vi "Pre Test Konfig.vi"() -> ()   [LabVIEW 2020, in "EPA 1065.lvlib" / "Pre-test verification 1065-520.lvlib"]
uses:
  Pre-test verification 1065-520.lvlib
  Allgemein/allgemeine Sub-VIs.lvlib
  Seiten/FT-IR/FT-IR.lvlib
  Seiten/FT-IR/FGV FT-IR Gasliste Aktionen.ctl
  Messdaten/Aktionen FGV Messdaten.ctl
  Messdaten/Messdaten.lvlib
  Seiten/Grafik/Grafik.lvlib
  Funktionstasten/Funktionstasten.lvlib
  Funktionstasten/Funktionstasten-Aktion.ctl
  Funktionstasten/Zustaende.ctl
  Seiten/Gaszuordnung AO/Gaszuordnung AO.lvlib
  Seiten/Gaszuordnung AO/FGV Gaszuordnung Grenzen&Einheit Aktion.ctl
  EPA 1065.lvlib
  Allgemeine VIs/Aktion Wertaenderung Gasliste.ctl
  Allgemeine VIs/Aktion Test Status.ctl
  Sprachverwaltung/Sprachverwaltung.lvlib
  Sprachverwaltung/FGV Aktion Tabelle zerlegen.ctl
  Aktion FGV Pre Test Daten.ctl
  Aktion FGV Pre Test Zustandsautomat.ctl
  PDF_Interface/PDF Interface Helper/PDFResultPictures.ctl
  PDF_Interface/PDF Interface Helper/PDF Interface Helper.lvlib
  T90 1065-308/Ergebnis.ctl
  T90 1065-308/T90 Test 1065-308.lvlib
  Visualisierungs Elemente/Zahlen-Ausgabefeld.ctl
  Pre Konfig Daten.ctl
  Modus Pre Test.ctl
panel:
  out "Ergebnis PDF FALSE":T1 caption="Ergebnis 2"
  out "Ergebnis PDF TRUE":T1 caption="Ergebnis 1"
  in  "Gasliste geändert":bool
  in  "Registerkarte":enum32{"Settings", "PRE Test", "Result"}(tab)
  in  "Pre Konfig Daten":T2={"Bearbeiter:"="", "Messgerät:"="", "Seriennummer:"="", "Modus"=0, "Pfad:"=path "D:/IAG_Data/Log", "Textname:"="", "N2 Aufschaltzeit:"=120.0, "Flow weighted mean:"=0.0} {"Flow weighted mean:" min=10.0; "N2 Aufschaltzeit:" min=10.0; "Modus" items=["Messen", "CalGas zu Entnahme"]}
  in  "Speichern":bool
  out "Einheit":string
  out "Komponente":string caption="Komponente:"
  out "Status":string
  out "Pre":waveform(dbl)(graph)
  in  "Test Start":bool
  in  "Abbrechen":bool
  out "Istwert":T4 caption="Istwert:" format="%.2f"
  out "Mwert":sgl format="%.3f"
  out "PMwert":sgl format="%.3f"
  out "Einheit Genauigkeit 2":string
  out "Ergebnis 1":T1
  out "Ergebnis THC":string
  out "Grenze":string caption="Grenzwert:"
  out "Einheit Genauigkeit":string
  out "Pre Result":waveform(dbl)(graph) caption="Pre"
  in  "Print PDF":bool caption="Abbrechen"
  out "Komponente 2":string caption="Komponente:"
  # "Pre Test Verification EPA CRF40 §1065.520"
  # "Allgemeine Einstellungen"
  # "Protokoll Einstellung"
  # "ppm"
  # "sec."
  # "±"
  # "x"
  # "Grenzwerte"
  # "Ergebnis"
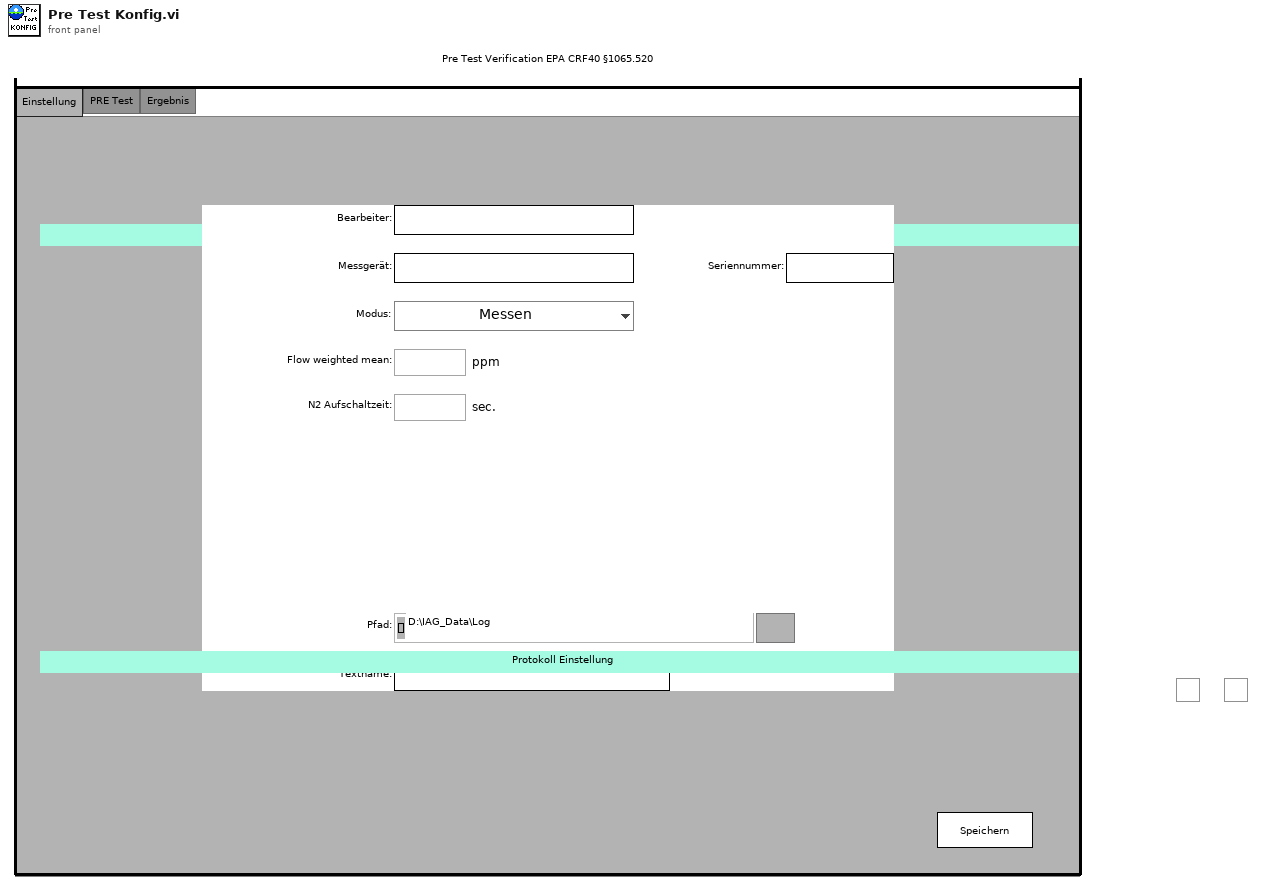
[diagram p1: front panel]
types:
  T1 = typedef "EPA 1065.lvlib/T90 Test 1065-308.lvlib/Ergebnis.ctl" = bool
  T2 = typedef "EPA 1065.lvlib/Pre-test verification 1065-520.lvlib/Pre Konfig Daten.ctl" = cluster{"Bearbeiter:":string, "Messgerät:":string, "Seriennummer:":string, "Modus":T3, "Pfad:":path, "Textname:":string, "N2 Aufschaltzeit:":dbl, "Flow weighted mean:":dbl}
  T3 = typedef "EPA 1065.lvlib/Pre-test verification 1065-520.lvlib/Modus Pre Test.ctl" = u16
  T4 = typedef "Zahlen-Ausgabefeld.ctl" = sgl
  T5 = typedef "EPA 1065.lvlib/Pre-test verification 1065-520.lvlib/Aktion FGV Pre Test Daten.ctl" = enum16{"lesen", "Konfig Daten", "PDF einstellen", "laden", "speichern", "Werte schreiben", "Auswerten"}
  T6 = typedef "EPA 1065.lvlib/Pre-test verification 1065-520.lvlib/Aktion FGV Pre Test Zustandsautomat.ctl" = enum16{"init", "lesen", "leerlauf", "0-Gas aufschalten", "0-Gas abwarten", "aufzeichnen", "fertig", "abbrechen"}
  T7 = typedef "Gaszuordnung AO.lvlib/FGV Gaszuordnung Grenzen&Einheit Aktion.ctl" = enum16{"Lesen", "Schreiben Min", "Schreiben Max", "Laden", "Speichern"}
  T8 = typedef "FT-IR.lvlib/FGV FT-IR Gasliste Aktionen.ctl" = enum16{"lesen", "Gasliste FT-IR", "Gasliste ausgelesen", "laden", "speichern", "löschen"}
  T9 = typedef "Sprachverwaltung.lvlib/FGV Aktion Tabelle zerlegen.ctl" = enum16{"laden", "vereinzeln", "speichern"}
  T10 = typedef "Messdaten.lvlib/Aktionen FGV Messdaten.ctl" = enum16{"lesen", "schreiben", "löschen", "Mittelwerte", "Komponente"}
  T11 = typedef "PDF Interface.lvlib/PDF Interface Helper.lvlib/PDFResultPictures.ctl" = cluster{"Yes Ctl Refnum":refnum<vi>, "No Ctl Refnum":refnum<vi>}
  T12 = typedef "String - Ausgabefeld.ctl" = string
  T13 = typedef "EPA 1065.lvlib/Aktion Wertaenderung Gasliste.ctl" = enum16{"Init", "lesen", "Gasliste geändert", "ARN inaktiv", "LEAK inaktiv", "Interference 366 inaktiv", "T90 inaktiv", "Interference 375 inaktiv", "Chiller inaktiv", "FID O2 inaktiv", "FID Opti inaktiv", "Drift inaktiv", "Pre Test inaktiv", "LinV2 inaktiv", "HovaCAL Interference inaktiv"}
  T14 = typedef "EPA 1065.lvlib/Aktion Test Status.ctl" = enum16{"init", "lesen", "prüfen", "Interference 366", "Interference 375", "Chiller läuft", "Drift läuft", "Pre Test läuft", "FID Optimization läuft", "FID Interference läuft", "HovaCAL Interference", "LinV2"}
  T15 = typedef "Funktionstasten.lvlib/Zustaende.ctl" = enum16{"Standby", "Pause", "Eco", "Messen", "Kalibrieren", "Spülen Filter", "Spülen Leitung", "Umgebungsluft", "0-Gas", "Cal-Gas", "CG zu PNS", "-------------", "Init 1", "Init 2", "Init 3", "Init 4", "Messen vorbereiten", "Messen durchführen", "Exit"}
  T16 = typedef "Funktionstasten.lvlib/Funktionstasten-Aktion.ctl" = enum16{"Initialisieren", "Zustand setzen", "Taste gedrückt", "Fehler speichern", "Lesen", "Manuell", "Remote", "Bitparallel", "Samplepoint", "Zeit Prüfen", "reset Umschalten"}
  T17 = typedef "EPA 1065.lvlib/Pre-test verification 1065-520.lvlib/Pre Werte.ctl" = cluster{"THC Wert":dbl, "Berechnetes Limit":dbl, "Bestanden":bool}
  T18 = typedef "EPA 1065.lvlib/Aktive Tests Cluster.ctl" = cluster{"ANR läuft":bool, "T90 läuft":bool, "Leak läuft":bool, "Interference 366 läuft":bool, "Interference 375 läuft":bool, "Chiller läuft":bool, "FID Interference läuft":bool, "FID optimization läuft":bool, "Drift läuft":bool, "Pre-test läuft":bool, "HovaCAL Interference läuft":bool, "LinV2 läuft":bool}
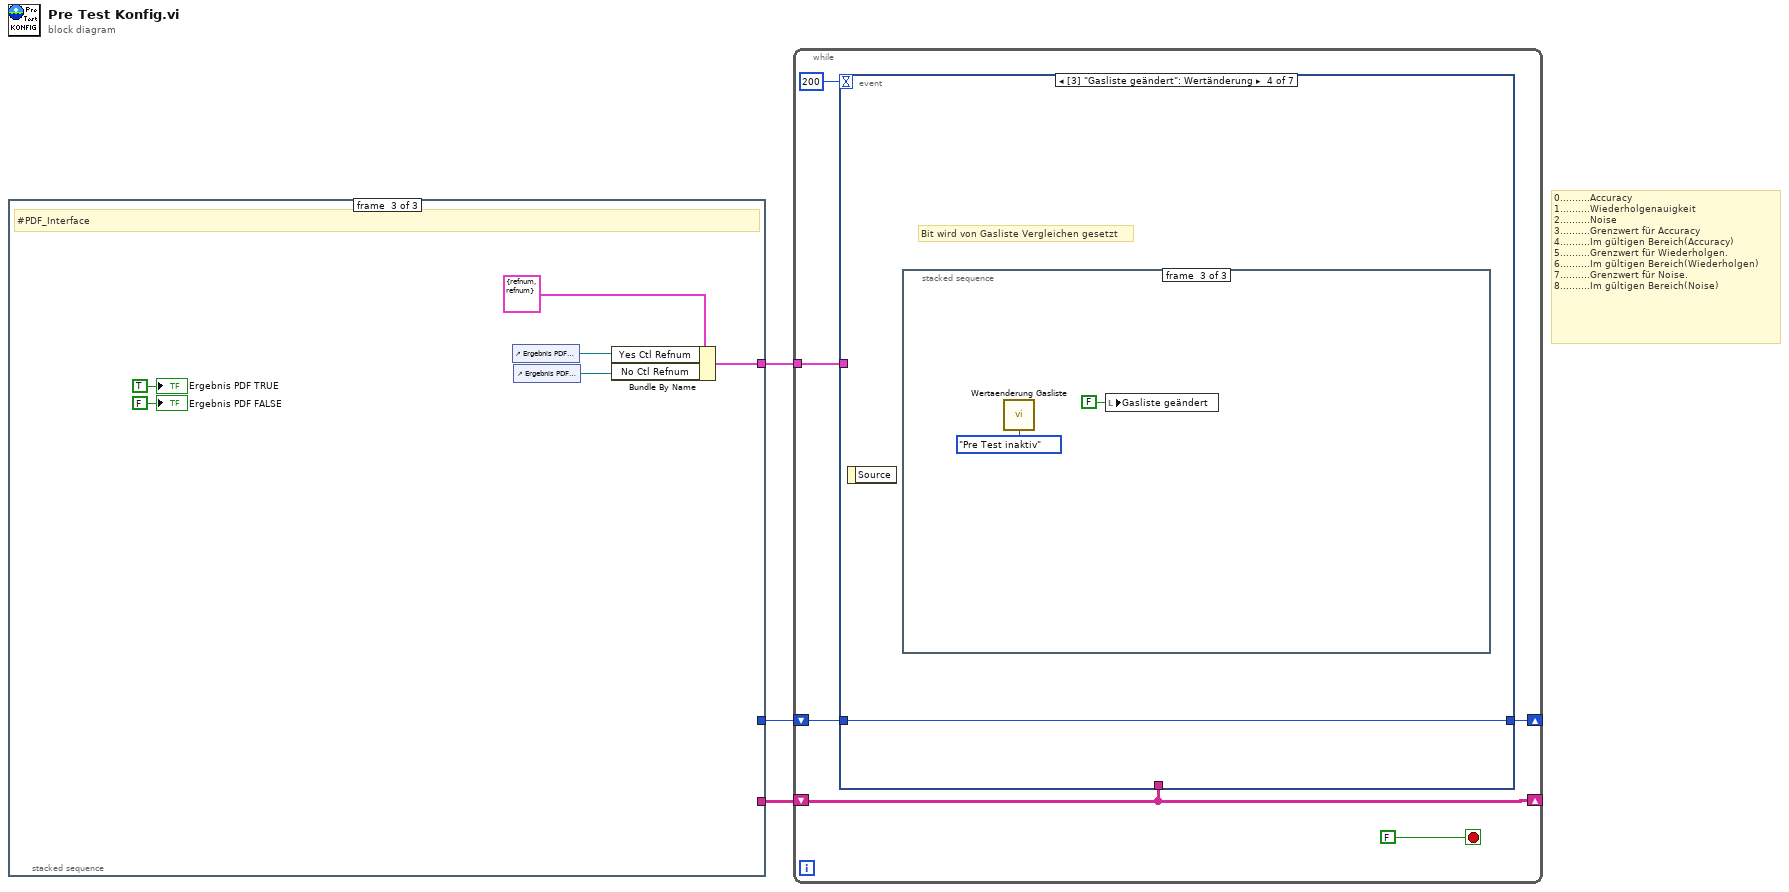
[diagram p0: block diagram]
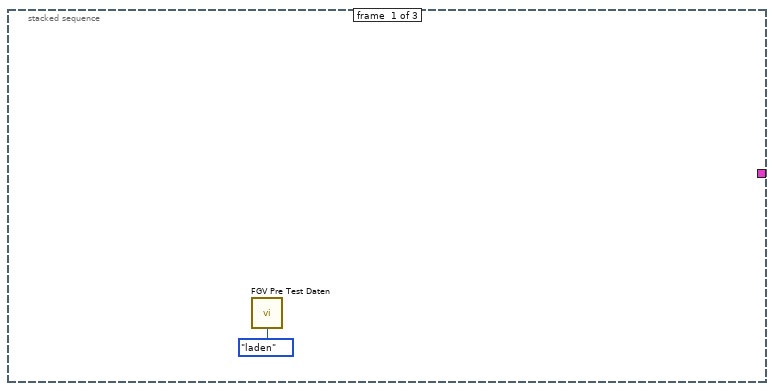
[diagram p2: hidden frame]
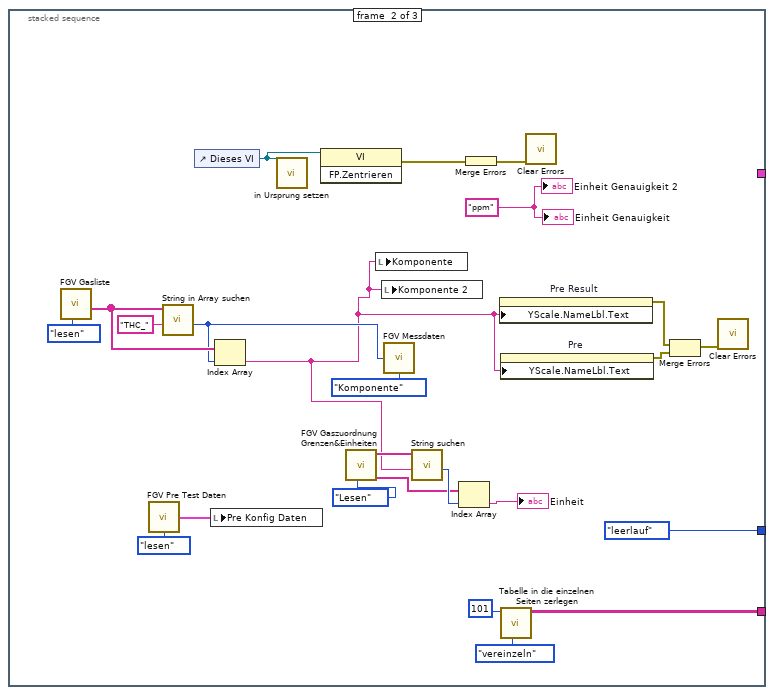
[diagram p3: hidden frame]
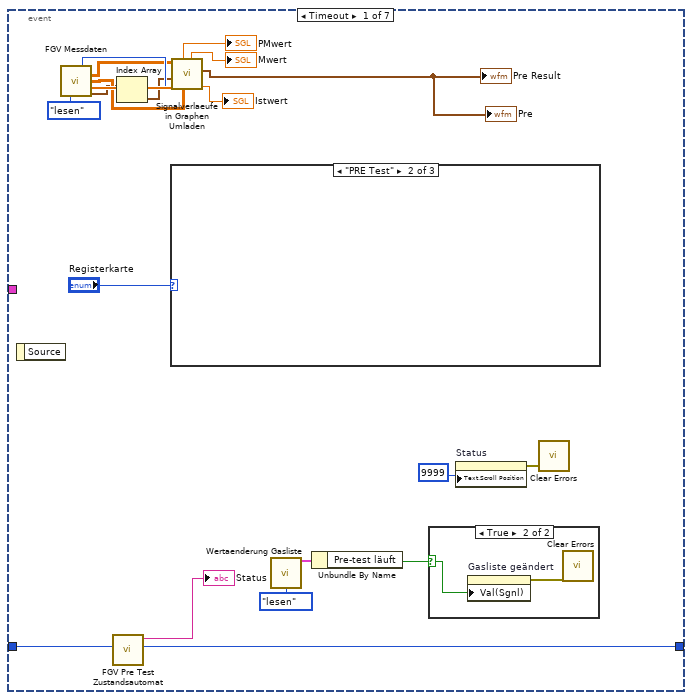
[diagram p4: hidden frame]
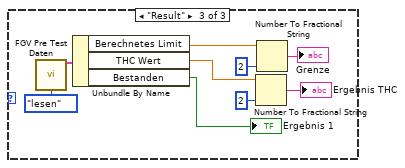
[diagram p6: hidden frame]
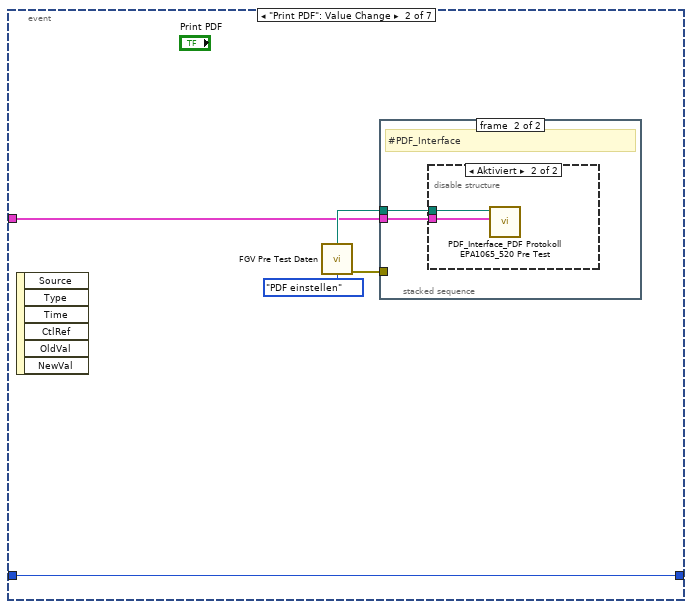
[diagram p8: hidden frame]
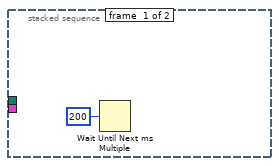
[diagram p9: hidden frame]
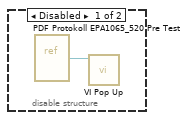
[diagram p10: hidden frame]
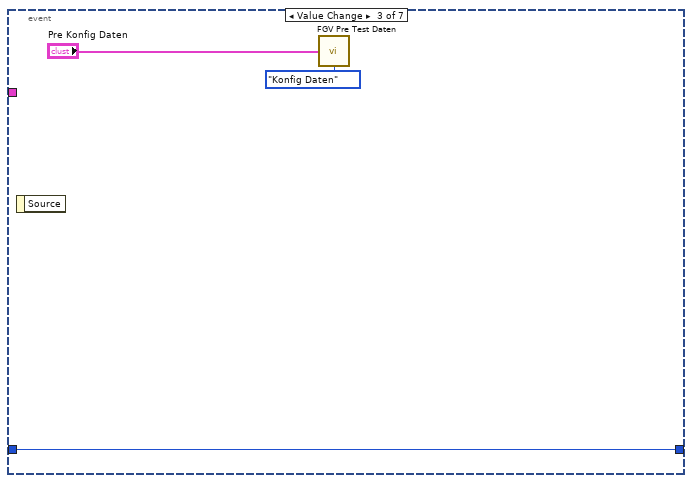
[diagram p11: hidden frame]
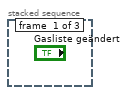
[diagram p12: hidden frame]
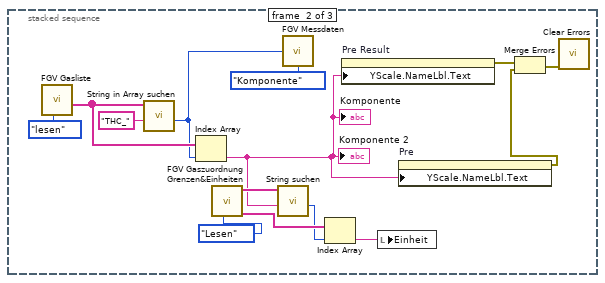
[diagram p13: hidden frame]
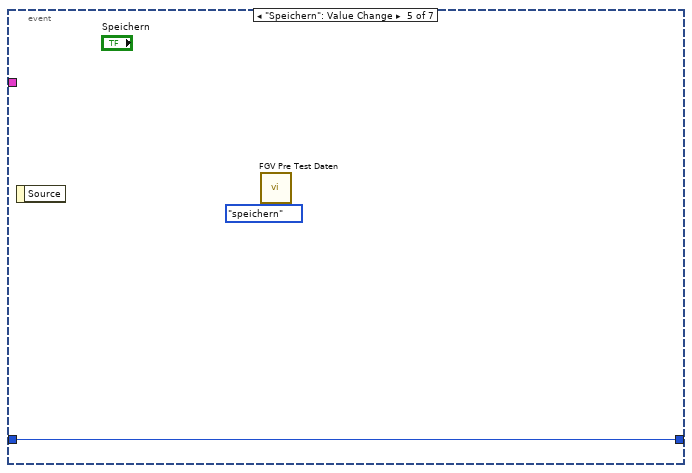
[diagram p14: hidden frame]
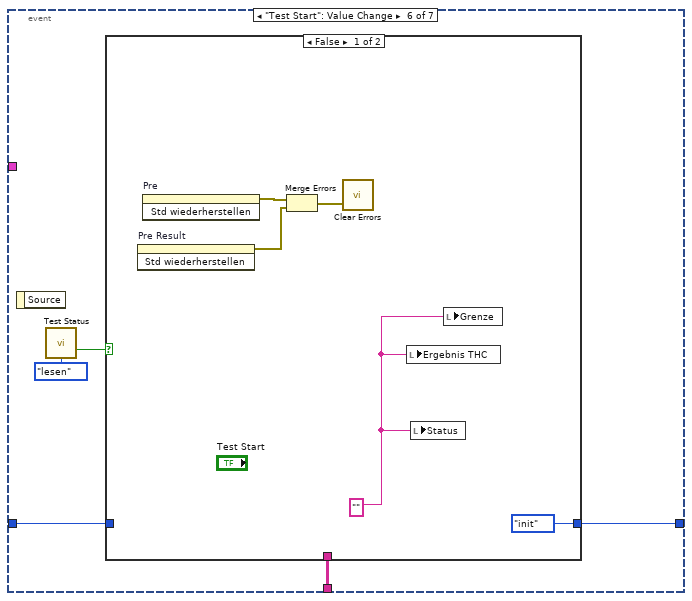
[diagram p15: hidden frame]
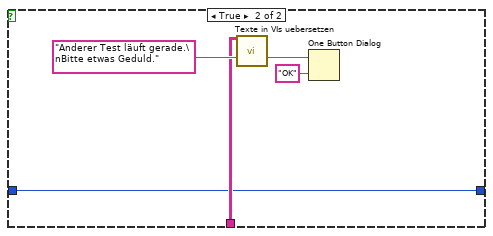
[diagram p16: hidden frame]
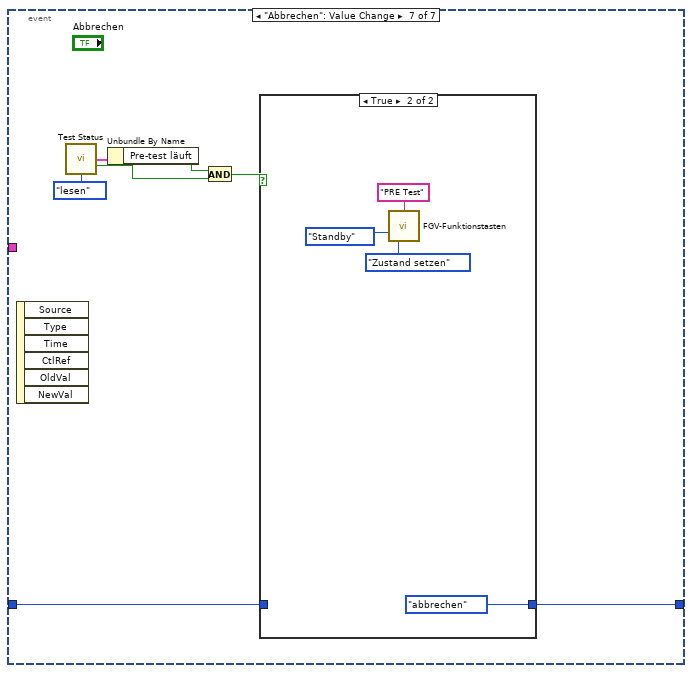
[diagram p17: hidden frame]
diagram:
  # "0..........Accuracy\n1..........Wiederholgenauigkeit\n2..........Noise\n3..........Grenzwert für Accuracy\n4..........Im gültigen Bereich(Accuracy)\n5..........Grenzwert für Wiederholgen.\n6..........Im gültigen Bereich(Wiederholgen)\n7..........Grenzwert für Noise.\n8..........Im gültigen Bereich(Noise)"
  n1 = stacked-sequence {
    tunnel: [_ w22 _] -> w3
    tunnel: [_ Aktion_FGV_Pre_Test_Zustandsautomat."leerlauf" ("Aktion") _] -> w2
    tunnel: [_ _ w29] -> w1
    frame #0 {
      n2 = call "FGV Pre Test Daten.vi"("Aktion"=Aktion_FGV_Pre_Test_Daten."laden") -> ()  [unwired: 11 in, 4 out]
    }
    frame #1 {
      w21 = "ppm" ("Einheit Genauigkeit 2")
      n3 = call "FGV Gasliste.vi"("Aktionen"=FGV_FT-IR_Gasliste_Aktionen."lesen") -> ("Aktuelle Gasliste gesamt"=w16:T12[])  [unwired: 8 in, 2 out]
      n4 = call "FGV Pre Test Daten.vi"("Aktion"=Aktion_FGV_Pre_Test_Daten."lesen") -> ("T90 Konfig Daten 2"=w19:T2)  [unwired: 11 in, 3 out]
      n5 = call "String in Array suchen.vi"("Nach String/Zeichen suchen (-)"="THC_", "String-Array"=w16) -> ("Index"=w15:i32)  [unwired: 7 in, 2 out]
      n6 = control-ref of="Dieses VI"() -> (w26:refnum<vi>)
      n7 = local write "Pre Konfig Daten"(w19) -> ()
      n8 = Index Array(array=w16, index=w15) -> (element=w8:T12)
      n9 = call "in Ursprung setzen.vi"("VI Referenz"=w26) -> ()  [unwired: 10 in, 1 out]
      n10 = invoke class="VI" method="FP.Zentrieren"(reference=w26) -> (error out=w25:errorcluster)  [unwired: 2 in, 2 out]
      n11 = call "FGV Gaszuordnung Grenzen&Einheiten.vi"("Aktion"=FGV_Gaszuordnung_Grenzen&Einheit_Aktion."Lesen") -> ("Einheit neu"=w11:string[], "Namen neu"=w12:string[])  [unwired: 7 in, 2 out]
      n12 = local write "Komponente"(w8) -> ()
      n13 = local write "Komponente 2"(w8) -> ()
      n14 = call "FGV Messdaten.vi"("Komponente"=w15, "Aktionen"=Aktionen_FGV_Messdaten."Komponente") -> ()  [unwired: 5 in, 9 out]
      n15 = call "String suchen.vi"("Gasname"=w8, "Such-Namen"=w12) -> ("Index"=w13:i32)  [unwired: 8 in, 1 out]
      n16 = Index Array(array=w11, index=w13) -> (element=→"Einheit":string)
      n17 = Merge Errors(w25) -> (w27:errorcluster)
      n18 = property on="Pre Result" class="SVGraph (strikt)"("YScale.NameLbl.Text"=w8) -> (error out=w6:errorcluster)  [unwired: 2 in, 1 out]
      n19 = property on="Pre" class="SVGraph (strikt)"("YScale.NameLbl.Text"=w8) -> (error out=w7:errorcluster)  [unwired: 2 in, 1 out]
      n20 = call "Tabelle in die einzelnen Seiten zerlegen.vi"("Aktion"=FGV_Aktion_Tabelle_zerlegen."vereinzeln", "Index (Seite)"=101) -> ("Sprachliste"=w22:string[][])  [unwired: 7 in, 2 out]
      n21 = call <vilib>:"Clear Errors.vi"("error in (no error)"=w27) -> ()  [unwired: 5 in, 2 out]
      n22 = Merge Errors(w6, w7) -> (w5:errorcluster)
      n23 = call <vilib>:"Clear Errors.vi"("error in (no error)"=w5) -> ()  [unwired: 5 in, 2 out]
      "Einheit Genauigkeit" <- w21
      "Einheit Genauigkeit 2" <- w21
    }
    frame #2 {
      # "#PDF_Interface"
      n24 = control-ref of="Ergebnis PDF TRUE"() -> (w31:refnum<vi>)
      n25 = control-ref of="Ergebnis PDF FALSE"() -> (w30:refnum<vi>)
      n26 = Bundle By Name(cluster=T11 {"Yes Ctl Refnum"=refnum, "No Ctl Refnum"=refnum} ("ResultPictures"), "Yes Ctl Refnum"=w31, "No Ctl Refnum"=w30) -> (w29:T11)
      "Ergebnis PDF TRUE" <- T1 TRUE ("Ergebnis PDF TRUE")
      "Ergebnis PDF FALSE" <- T1 FALSE ("Ergebnis PDF FALSE")
    }
  }
  n27 = while {
    shift-right: [w38] -> _
    shift-left: w3 -> [w38]
    shift-right: [w36] -> _
    shift-left: w2 -> [w37]
    tunnel: w1 -> [w35]
    stop <- FALSE stop-if-true
    n28 = event shown="[3] \"Gasliste geändert\": Wertänderung" {
      selector: _ -> [_ _ _ _ _ _ _]
      dyn-events: _ -> [_ _ _ _ _ _ _]
      timeout: 200 -> [_ _ _ _ _ _ _]
      tunnel: w38 -> [_ _ _ _ _ w107 _]
      tunnel: w37 -> [w45 w76 w83 w86 w103 w105 w120]
      tunnel: [w44 w76 w83 w86 w103 w106 w121] -> w36
      tunnel: w35 -> [_ w72 _ _ _ _ _]
      event Timeout {
        n29 = event-data() -> ()  [unwired: 1 in, 1 out]
        n30 = call "FGV Messdaten.vi"("Aktionen"=Aktionen_FGV_Messdaten."lesen") -> ("Komponente"=w58:u16, "Messdaten"=w55:sgl[][], "Mittelwertdaten"=w59:sgl[][], "Deviation"=w60:sgl[], "Zeitstempeln"=w53:timestamp[])  [unwired: 6 in, 4 out]
        n31 = call "FGV Pre Test Zustandsautomat.vi"("Aktion"=w45) -> ("Aktion"=w44:T6, "Status"=→"Status":string)  [unwired: 7 in, 2 out]
        n32 = Index Array(array=w53) -> (element=w54:timestamp)  [unwired: 1 in]
        n33 = case shown="\"PRE Test\"" "Registerkarte" {
          frame "Settings", Default {
          }
          frame "PRE Test" {
          }
          frame "Result" {
            n34 = call "FGV Pre Test Daten.vi"("Aktion"=Aktion_FGV_Pre_Test_Daten."lesen") -> ("Daten/Ergebnisse"=w68:T17)  [unwired: 11 in, 3 out]
            n35 = Unbundle By Name(w68) -> ("Berechnetes Limit"=w62:dbl, "THC Wert"=w67:dbl, "Bestanden"=→"Ergebnis 1":bool)
            n36 = Number To Fractional String(number=w67, precision (6)=i16 2 ("Genauigkeit (6)")) -> (F-format string=→"Ergebnis THC":string)  [unwired: 2 in]
            n37 = Number To Fractional String(number=w62, precision (6)=i16 2 ("Genauigkeit (6)")) -> (F-format string=→"Grenze":string)  [unwired: 2 in]
          }
        }
        n38 = call "Signalverlaeufe in Graphen Umladen.vi"("Deviation"=w60, "Mittelwertdaten"=w59, "Gas-Auswahl"=w58, "t0"=w54, "Werte"=w55) -> ("Konzentration"=→"Istwert":sgl, "Mittelwert"=→"Pre Result" →"Pre":waveform(dbl), "aktuelle Mittelwert"=→"Mwert":sgl, "Deviation"=→"PMwert":sgl)  [unwired: 2 in, 1 out]
        n39 = call "Wertaenderung Gasliste.vi"("Aktion"=Aktion_Wertaenderung_Gasliste."lesen") -> ("Tests"=w47:T18)  [unwired: 13 in, 1 out]
        n40 = Unbundle By Name(w47) -> ("Pre-test läuft"=w41:bool)
        n41 = case shown="True" w41 {
          selector: w41 -> [_ w70]
          frame False {
          }
          frame True {
            n42 = property on="Gasliste geändert" class="Bool. (strikt)"("Val(Sgnl)"=w70) -> (error out=w71:errorcluster)  [unwired: 2 in, 1 out]
            n43 = call <vilib>:"Clear Errors.vi"("error in (no error)"=w71) -> ()  [unwired: 5 in, 2 out]
          }
        }
        n44 = property on="Status" class="Str"("Text.Scroll Position"=u32 9999 ("Text.Anzeigeposition")) -> (error out=w50:errorcluster)  [unwired: 2 in, 1 out]
        n45 = call <vilib>:"Clear Errors.vi"("error in (no error)"=w50) -> ()  [unwired: 5 in, 2 out]
      }
      event "Print PDF": Value Change {
        n46 = event-data() -> ()  [unwired: 1 in, 6 out]
        n47 = call "FGV Pre Test Daten.vi"("Aktion"=Aktion_FGV_Pre_Test_Daten."PDF einstellen") -> ("PDF Pfad"=w73:path, "error out"=w74:errorcluster)  [unwired: 11 in, 2 out]
        n48 = stacked-sequence {
          tunnel: w74 -> [_ _]
          tunnel: w73 -> [_ w79]
          tunnel: w72 -> [_ w78]
          frame #0 {
            n49 = Wait Until Next ms Multiple(millisecond multiple=u32 200 ("ms")) -> ()  [unwired: 1 out]
          }
          frame #1 {
            # "#PDF_Interface"
            n50 = disable-structure shown="Aktiviert" {
              disable-tunnel: w79 -> [_ w82]
              disable-tunnel: w78 -> [_ w81]
              frame Disabled {
                n51 = vi-ref "PDF Protokoll EPA1065_520 Pre Test.vi"() -> (w80:refnum<vi>)
                n52 = call "VI Pop Up.vi"("VI Referenz"=w80) -> ()  [unwired: 10 in, 1 out]
              }
              frame Enabled {
                n53 = call "PDF_Interface_PDF Protokoll EPA1065_520 Pre Test.vi"("ResultPictures"=w81, "Save PDF File Path"=w82) -> ()  [unwired: 9 in, 1 out]
              }
            }
          }
        }
      }
      event Value Change {
        n54 = event-data() -> ()  [unwired: 1 in, 1 out]
        n55 = call "FGV Pre Test Daten.vi"("T90 Konfig Daten"="Pre Konfig Daten", "Aktion"=Aktion_FGV_Pre_Test_Daten."Konfig Daten") -> ()  [unwired: 10 in, 4 out]
      }
      event "Gasliste geändert": Value Change {
        # "Bit wird von Gasliste Vergleichen gesetzt"
        n56 = event-data() -> ()  [unwired: 1 in, 1 out]
        n57 = stacked-sequence {
          frame #0 {
          }
          frame #1 {
            n58 = call "FGV Gasliste.vi"("Aktionen"=FGV_FT-IR_Gasliste_Aktionen."lesen") -> ("Aktuelle Gasliste gesamt"=w99:T12[])  [unwired: 8 in, 2 out]
            n59 = call "String in Array suchen.vi"("Nach String/Zeichen suchen (-)"="THC_", "String-Array"=w99) -> ("Index"=w96:i32)  [unwired: 7 in, 2 out]
            n60 = Index Array(array=w99, index=w96) -> (element=w90:T12)
            "Komponente" <- w90
            "Komponente 2" <- w90
            n61 = call "FGV Gaszuordnung Grenzen&Einheiten.vi"("Aktion"=FGV_Gaszuordnung_Grenzen&Einheit_Aktion."Lesen") -> ("Einheit neu"=w94:string[], "Namen neu"=w93:string[])  [unwired: 7 in, 2 out]
            n62 = call "String suchen.vi"("Gasname"=w90, "Such-Namen"=w93) -> ("Index"=w92:i32)  [unwired: 8 in, 1 out]
            n63 = call "FGV Messdaten.vi"("Komponente"=w96, "Aktionen"=Aktionen_FGV_Messdaten."Komponente") -> ()  [unwired: 5 in, 9 out]
            n64 = Index Array(array=w94, index=w92) -> (element=w91:string)
            n65 = property on="Pre Result" class="SVGraph (strikt)"("YScale.NameLbl.Text"=w90) -> (error out=w89:errorcluster)  [unwired: 2 in, 1 out]
            n66 = local write "Einheit"(w91) -> ()
            n67 = property on="Pre" class="SVGraph (strikt)"("YScale.NameLbl.Text"=w90) -> (error out=w87:errorcluster)  [unwired: 2 in, 1 out]
            n68 = Merge Errors(w89, w87) -> (w88:errorcluster)
            n69 = call <vilib>:"Clear Errors.vi"("error in (no error)"=w88) -> ()  [unwired: 5 in, 2 out]
          }
          frame #2 {
            n70 = call "Wertaenderung Gasliste.vi"("Aktion"=Aktion_Wertaenderung_Gasliste."Pre Test inaktiv") -> ()  [unwired: 13 in, 2 out]
            n71 = local write "Gasliste geändert"(FALSE ("Gasliste geändert")) -> ()
          }
        }
      }
      event "Speichern": Value Change {
        n72 = event-data() -> ()  [unwired: 1 in, 1 out]
        n73 = call "FGV Pre Test Daten.vi"("Aktion"=Aktion_FGV_Pre_Test_Daten."speichern") -> ()  [unwired: 11 in, 4 out]
      }
      event "Test Start": Value Change {
        n74 = event-data() -> ()  [unwired: 1 in, 1 out]
        n75 = call "Test Status.vi"("Aktion"=Aktion_Test_Status."lesen") -> ("Tests sperren"=w108:bool)  [unwired: 11 in, 3 out]
        n76 = case shown="False" w108 {
          tunnel: w107 -> [_ w116]
          tunnel: [Aktion_FGV_Pre_Test_Zustandsautomat."init" ("Aktion") w115] -> w106
          tunnel: w105 -> [_ w115]
          frame False {
            w111 = "" ("Status")
            n77 = invoke on="Pre Result" class="SVGraph (strikt)" method="Std wiederherstellen"() -> (error out=w112:errorcluster)  [unwired: 3 in, 2 out]
            n78 = invoke on="Pre" class="SVGraph (strikt)" method="Std wiederherstellen"() -> (error out=w113:errorcluster)  [unwired: 3 in, 2 out]
            n79 = Merge Errors(w113, w112) -> (w114:errorcluster)
            n80 = call <vilib>:"Clear Errors.vi"("error in (no error)"=w114) -> ()  [unwired: 5 in, 2 out]
            n81 = local write "Ergebnis THC"(w111) -> ()
            n82 = local write "Status"(w111) -> ()
            n83 = local write "Grenze"(w111) -> ()
          }
          frame True {
            n84 = call "Texte in VIs uebersetzen.vi"("Sprachliste"=w116, "String zum Übersetzen"="Anderer Test läuft gerade.\nBitte etwas Geduld." ("Nachricht")) -> ("String zum Übersetzen"=w117:string)  [unwired: 9 in, 4 out]
            n85 = One Button Dialog(message=w117, button name ("OK")="OK" ("Schaltflächentext (\"OK\")")) -> ()  [unwired: 1 out]
          }
        }
      }
      event "Abbrechen": Value Change {
        n86 = event-data() -> ()  [unwired: 1 in, 6 out]
        n87 = call "Test Status.vi"("Aktion"=Aktion_Test_Status."lesen") -> ("Aktive Tests"=w125:T18, "Tests sperren"=w123:bool)  [unwired: 11 in, 2 out]
        n88 = Unbundle By Name(w125) -> ("Pre-test läuft"=w124:bool)
        n89 = And(x=w124, y=w123) -> (x .and. y?=w122:bool)
        n90 = case shown="True" w122 {
          tunnel: [w127 Aktion_FGV_Pre_Test_Zustandsautomat."abbrechen" ("Aktion")] -> w121
          tunnel: w120 -> [w127 _]
          frame False {
          }
          frame True {
            n91 = call "FGV-Funktionstasten.vi"("Herkunft"="PRE Test", "Zustand"=Zustaende."Standby", "Aktion"=Funktionstasten-Aktion."Zustand setzen") -> ()  [unwired: 5 in, 8 out]
          }
        }
      }
    }
  }
